vi "Action Stop Pump.vi"(5 "Retry Attempts (0)":i32 min=0, 8 "error in":errorcluster, 11 "VISA resource name":refnum<visa-resource-name>) -> (0 "error out":errorcluster, 3 "VISA resource name out":refnum<visa-resource-name>)   [LabVIEW 2020, in "ChromTech Series III Pump.lvlib"]
doc: "Stop the pump."
uses:
  <instrlib>/ChromTech Series III Pump/ChromTech Series III Pump.lvlib
panel:
  out "Response":string
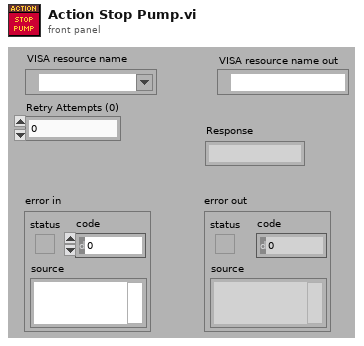
[diagram p1: front panel]
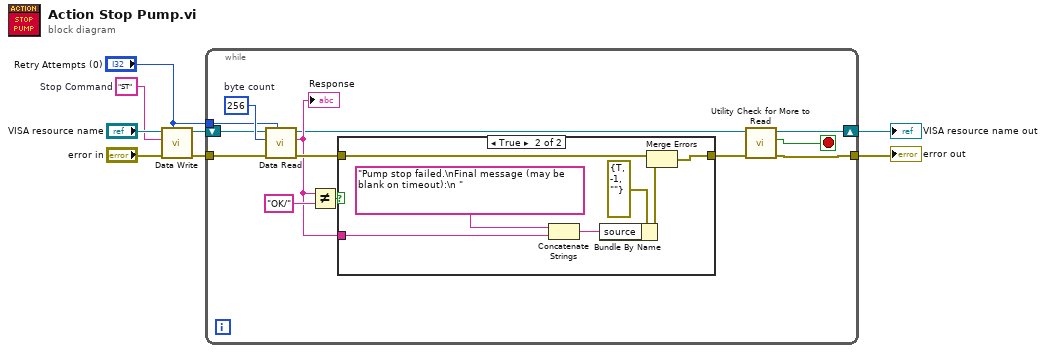
[diagram p0: block diagram]
diagram:
  w6 = "ST"  # Stop Command
  n1 = call <instrlib>:"Data Write.vi"("Retry Attempts (0)"="Retry Attempts (0)", "error in (no error)"="error in", "Command"=w6, "VISA Refnum in"="VISA resource name") -> ("error out"=w3:errorcluster, "VISA Refnum out"=w2:refnum<visa-resource-name>)  [unwired: 6 in]
  n2 = while {
    tunnel: "Retry Attempts (0)" -> [w14]
    shift-right: [w10] -> w4
    shift-left: w2 -> [w16]
    tunnel: w3 -> [w17]
    tunnel: [w12] -> w5
    stop <- w9 stop-if-true
    w21 = u32 256  # byte count
    n3 = call <instrlib>:"Data Read.vi"("Retry Attempts (0)"=w14, "error in (no error)"=w17, "Bytes to read"=w21, "VISA Refnum in"=w16) -> ("error out"=w18:errorcluster, "read buffer"=w15:string, "VISA Refnum out"=w11:refnum<visa-resource-name>)  [unwired: 5 in]
    "Response" <- w15
    n4 = Not Equal?(x=w15, y="OK/") -> (x != y?=w19:bool)
    n5 = case shown="True" w19 {
      tunnel: [w22 w28] -> w13
      tunnel: w18 -> [w22 w27]
      tunnel: w15 -> [_ w23]
      frame False {
      }
      frame True {
        n6 = Concatenate Strings("Pump stop failed.\nFinal message (may be blank on timeout):\n ", w23) -> (w25:string)
        n7 = Bundle By Name(cluster=errorcluster {"status"=TRUE, "code"=-1, "source"=""} ("error out"), "source"=w25) -> (w26:errorcluster)
        n8 = Merge Errors(w27, w26) -> (w28:errorcluster)
      }
    }
    n9 = call <instrlib>:"Utility Check for More to Read.vi"("error in (no error)"=w13, "VISA Refnum in"=w11) -> ("error out (unchanged)"=w12:errorcluster, "More to read?"=w9:bool, "VISA Refnum out"=w10:refnum<visa-resource-name>)  [unwired: 7 in]
  }
  "VISA resource name out" <- w4
  "error out" <- w5
